vi "SIRStrip.vi"(7 "lower h of strip":dbl format="%.2f", 8 "P":cluster{"x":dbl, "y":dbl, "z":dbl}={"x"=1.0, "y"=-5.0, "z"=1.0} {"x" format="%.2f"; "z" format="%.2f"; "y" format="%.2f"}, 9 "Variables":T1={"sound spd (cm/s)"=150000, "time step (s)"=1e-09} {"time step (s)" format="%.2e"}, 11 "strip":cluster{"Radius":dbl, "h":dbl, "a":dbl}={"Radius"=10.0, "h"=3.0, "a"=5.0} {"Radius" format="%.2f"; "a" format="%.2f"; "h" format="%.2f"}) -> (1 "lower":dbl[](graph), 2 "upper":dbl[](graph), 3 "h out":dbl[](graph), 4 "delay out":i32)   [LabVIEW 2022 SP3]
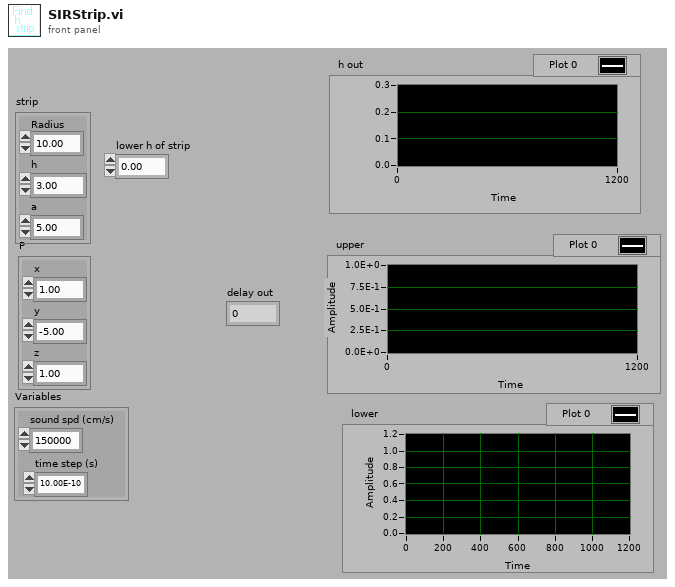
[diagram p1: front panel]
types:
  T1 = cluster{"sound spd (cm/s)":i32, "time step (s)":sgl}
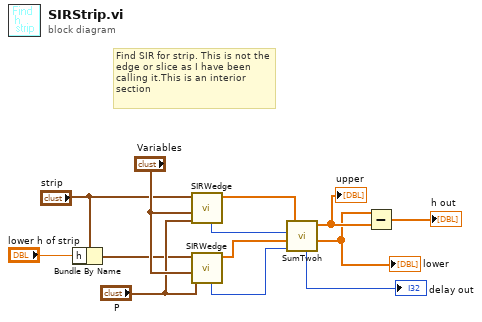
[diagram p0: block diagram]
diagram:
  # "Find SIR for strip. This is not the edge or slice as I have been calling it.This is an interior section"
  n1 = Bundle By Name(cluster="strip", "h"="lower h of strip") -> (w9:cluster{"Radius":dbl, "h":dbl, "a":dbl})
  n2 = call "SIRWedge.vi"("P"="P", "Variables"="Variables", "strip"="strip") -> ("h wedge"=w6:dbl[], "wedge delay"=w8:i32)  [unwired: 7 out]
  n3 = call "SIRWedge.vi"("P"="P", "Variables"="Variables", "strip"=w9) -> ("h wedge"=w5:dbl[], "wedge delay"=w7:i32)  [unwired: 7 out]
  n4 = call "SumTwoh.vi"("h1"=w6, "delay1"=w8, "h2"=w5, "delay2"=w7) -> ("delay out"=→"delay out":i32, "upper"=w2:dbl[], "lower"=w1:dbl[])  [unwired: 2 out]
  "lower" <- w1
  "upper" <- w2
  n5 = Subtract(x=w1, y=w2) -> (x-y=→"h out":dbl[])
